vi "Levelmeter_Split_Cluster.vi"(0 "Mischer Levelmeter":T2={"Plot"=[], "N-Shield (%)"=0.0, "He (%)"=0.0, "Coldtrap (%)"=0.0, "He - POT (%)"=0.0, "N-Shield Refill"=FALSE, "Last fill Shield"="", "Auto Refill Shield"=TRUE, "Trap Refill"=FALSE, "Last fill Coldtrap"="", "Auto Refill Trap"=TRUE, "Shield Refill"=FALSE, "Coldtrap Refill"=FALSE, "Auto Trap activatet"=FALSE, "Auto Shield Activatet"=FALSE}) -> (1 "Mischer Levelmeter Status":T3, 2 "Mischer Levelmeter  Control":T1={"N-Shield Refill"=FALSE, "Automatic Refill Shield"=TRUE, "Trap Refill"=FALSE, "Automatic Refill Trap"=TRUE})   [LabVIEW 2019]
uses:
  Mischer/Mischer_Levelmeter_Status.ctl
  Mischer/Mischer_Levelmeter-Cluster.ctl
  Mischer/Mischer_Levelmeter_Control.ctl
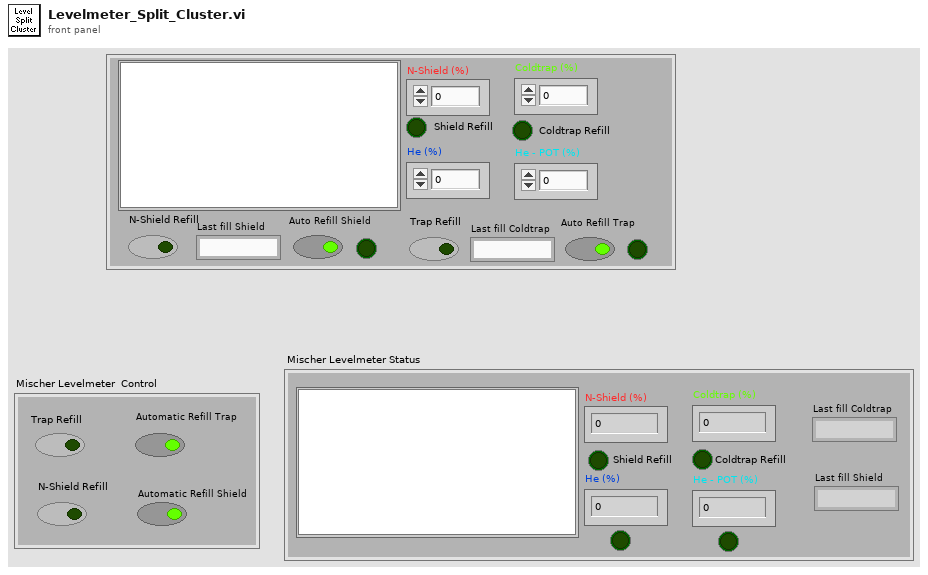
[diagram p1: front panel]
types:
  T1 = typedef "Mischer_Levelmeter_Control.ctl" = cluster{"N-Shield Refill":bool, "Automatic Refill Shield":bool, "Trap Refill":bool, "Automatic Refill Trap":bool}
  T2 = typedef "Mischer_Levelmeter-Cluster.ctl" = cluster{"Plot":dbl[][], "N-Shield (%)":dbl, "He (%)":dbl, "Coldtrap (%)":dbl, "He - POT (%)":dbl, "N-Shield Refill":bool, "Last fill Shield":string, "Auto Refill Shield":bool, "Trap Refill":bool, "Last fill Coldtrap":string, "Auto Refill Trap":bool, "Shield Refill":bool, "Coldtrap Refill":bool, "Auto Trap activatet":bool, "Auto Shield Activatet":bool}
  T3 = typedef "Mischer_Levelmeter_Status.ctl" = cluster{"Plot":dbl[][], "N-Shield (%)":dbl, "He (%)":dbl, "Coldtrap (%)":dbl, "He - POT (%)":dbl, "Shield Refill":bool, "Coldtrap Refill":bool, "Last fill Shield":string, "Last fill Coldtrap":string, "Auto Shield refill Activatet":bool, "Auto Trap refill activatet":bool}
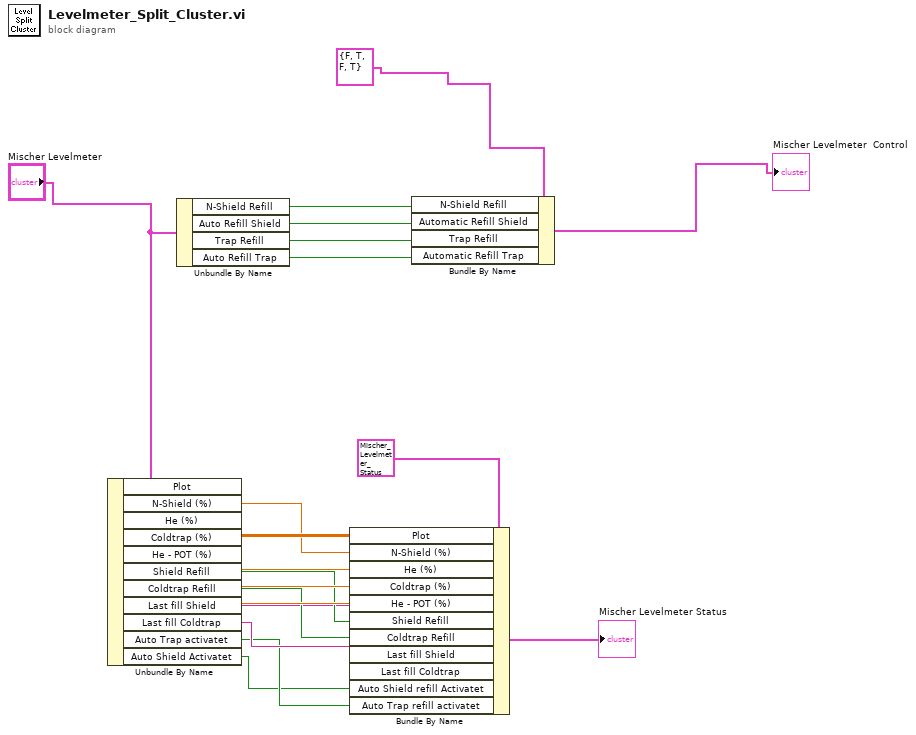
[diagram p0: block diagram]
diagram:
  n1 = Unbundle By Name("Mischer Levelmeter") -> ("Plot"=w18:dbl[][], "N-Shield (%)"=w17:dbl, "He (%)"=w16:dbl, "Coldtrap (%)"=w15:dbl, "He - POT (%)"=w14:dbl, "Shield Refill"=w6:bool, "Coldtrap Refill"=w5:bool, "Last fill Shield"=w4:string, "Last fill Coldtrap"=w3:string, "Auto Trap activatet"=w2:bool, "Auto Shield Activatet"=w1:bool)
  n2 = Unbundle By Name("Mischer Levelmeter") -> ("N-Shield Refill"=w10:bool, "Auto Refill Shield"=w9:bool, "Trap Refill"=w8:bool, "Auto Refill Trap"=w7:bool)
  n3 = Bundle By Name(cluster=T3 {"Plot"=[], "N-Shield (%)"=0.0, "He (%)"=0.0, "Coldtrap (%)"=0.0, "He - POT (%)"=0.0, "Shield Refill"=FALSE, "Coldtrap Refill"=FALSE, "Last fill Shield"="", "Last fill Coldtrap"="", "Auto Shield refill Activatet"=FALSE, "Auto Trap refill activatet"=FALSE} ("Mischer Levelmeter Status 2"), "Plot"=w18, "N-Shield (%)"=w17, "He (%)"=w16, "Coldtrap (%)"=w15, "He - POT (%)"=w14, "Shield Refill"=w6, "Coldtrap Refill"=w5, "Last fill Shield"=w4, "Last fill Coldtrap"=w3, "Auto Shield refill Activatet"=w1, "Auto Trap refill activatet"=w2) -> (→"Mischer Levelmeter Status":T3)
  n4 = Bundle By Name(cluster=T1 {"N-Shield Refill"=FALSE, "Automatic Refill Shield"=TRUE, "Trap Refill"=FALSE, "Automatic Refill Trap"=TRUE} ("Mischer Levelmeter  Control 2"), "N-Shield Refill"=w10, "Automatic Refill Shield"=w9, "Trap Refill"=w8, "Automatic Refill Trap"=w7) -> (→"Mischer Levelmeter  Control":T1)
